vi "Lorentzian function normal.vi"(3 "output control":T1, 4 "data":variant, 5 "X":dbl[](array[numeric]), 6 "params":dbl[](array[numeric])) -> (0 "error out":errorcluster, 1 "f'(X,a)":dbl[][](array[numeric]), 2 "f(X,a)":dbl[](array[numeric]))   [LabVIEW 2015]
doc: "Given a set of x-values and parameters (x0, gamma), outputs the resulting Lorentzian curve.\n\n(Connector panel is in a form that allows this VI to be passed to the Nonlinear Curve Fit.vi.)"
uses:
  <vilib>/gmath/NumericalOptimization/LM_output select.ctl
  <vilib>/gmath/NI_Gmath.lvlib
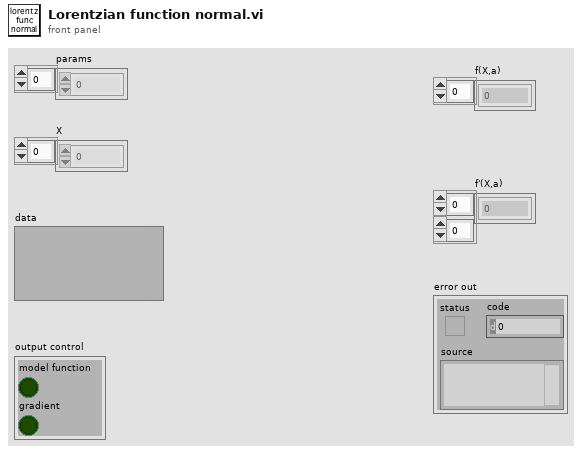
[diagram p1: front panel]
types:
  T1 = typedef "NI_Gmath.lvlib/LM_output select.ctl" = cluster{"model function":bool, "gradient":bool}
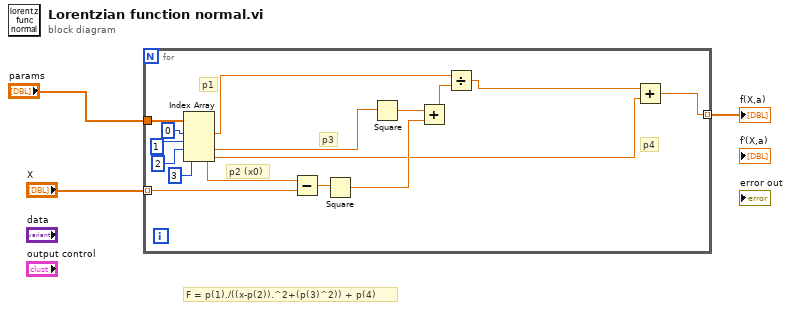
[diagram p0: block diagram]
diagram:
  # "F = p(1)./((x-p(2)).^2+(p(3)^2)) + p(4)"
  n1 = for {
    tunnel: "params" -> [w15]
    tunnel: "X" -> [w14] mode=indexing
    tunnel: [w7] -> w1 mode=indexing
    # "p3"
    # "p4"
    # "p2 (x0)"
    # "p1"
    n2 = Index Array(array=w15, index #1=0 ("index (col)"), index #2=1 ("disabled index (col)"), index #3=2 ("index"), index #4=3 ("index")) -> (element #1=w9:dbl, element #2=w16:dbl, element #3=w6:dbl, element #4=w8:dbl)
    n3 = Subtract(x=w16, y=w14) -> (x-y=w19:dbl)
    n4 = Square(x=w19) -> (x^2=w17:dbl)
    n5 = Square(x=w6) -> (x^2=w18:dbl)
    n6 = Add(x=w18, y=w17) -> (x+y=w5:dbl)
    n7 = Divide(x=w9, y=w5) -> (x/y=w4:dbl)
    n8 = Add(x=w4, y=w8) -> (x+y=w7:dbl)
  }
  "f(X,a)" <- w1
